vi "ModelCheckNew.vi"(8 "error in (no error)":errorcluster, 9 "ReScanNG":i32, 11 "Data In":T2) -> (0 "error out":errorcluster, 1 "States":T1=enum."Initialize", 2 "ReScanNG":i32, 3 "Data Out":T2)   [LabVIEW 2014]
uses:
  controls/Data1.ctl
  controls/Payjson.ctl
  controls/State.ctl
panel:
  out "Array 2":i32[](array[numeric])
  out "subarray":string[](array[string])
  out "logical AND":bool
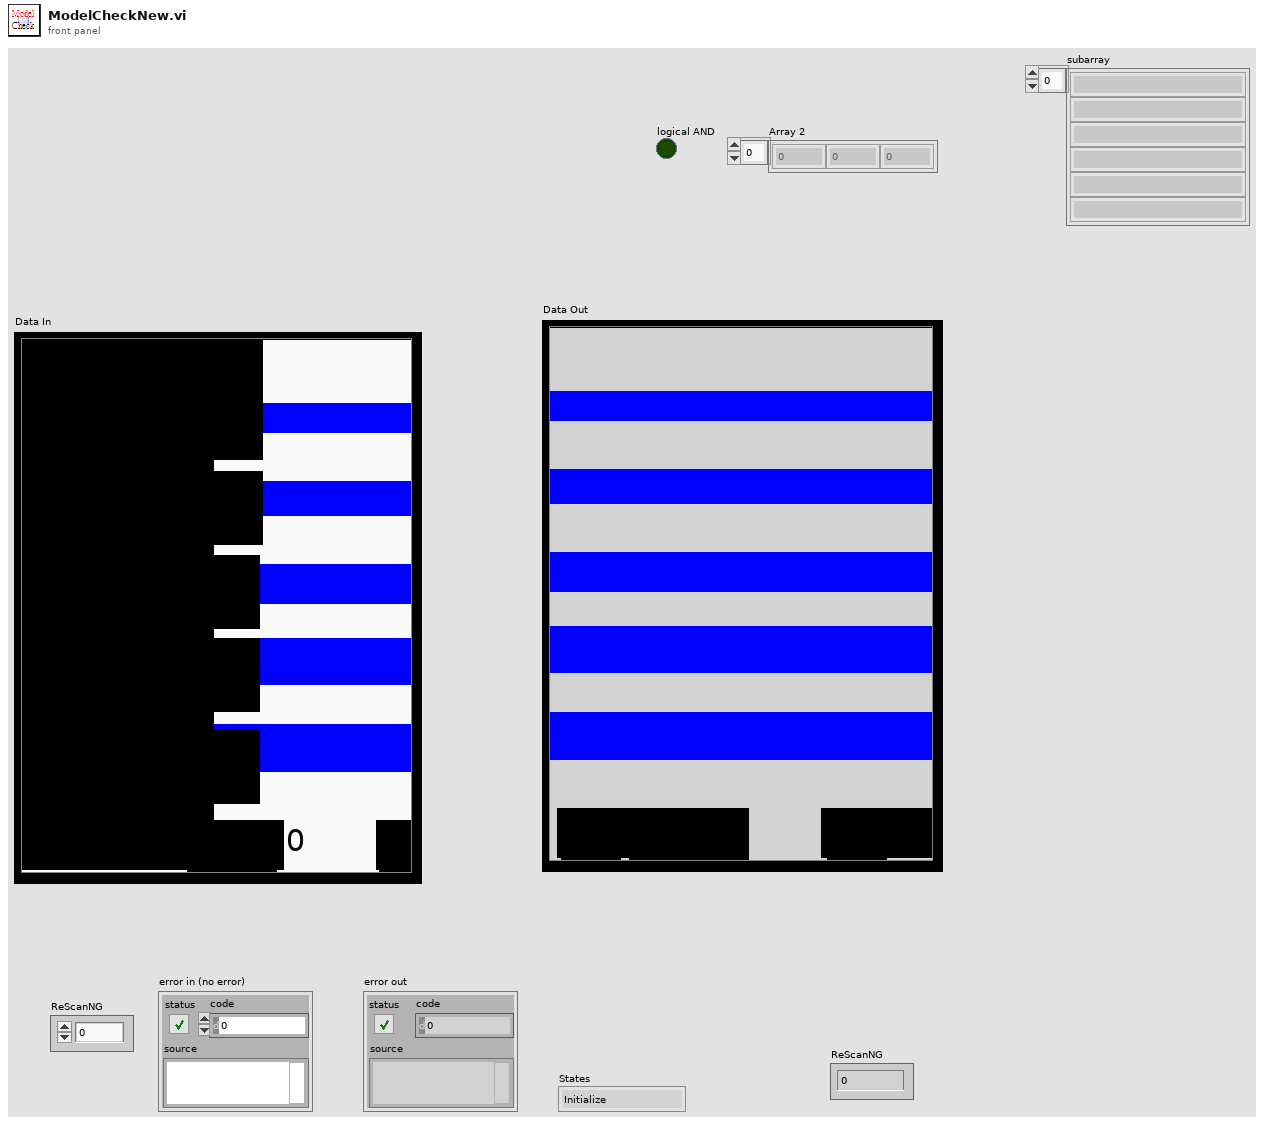
[diagram p1: front panel]
types:
  T1 = typedef "State.ctl" = enum16{"int", "Initalize0", "Initialize", "Wait for Scan", "State 1", "State 2", "NG", "NG1", "OK", "OKNG", "OKNG1", "Exit"}
  T2 = typedef "Data1.ctl" = cluster{"Date":string, "BarCode1":string, "BarCode2":string, "BarCode3":string, "Message":string, "OK Count":u16, "NG Count":u16, "Total Count":u16, "ModelData":string[][], "OK&NG":bool, "COM1":refnum<visa-resource-name>, "COM2":refnum<visa-resource-name>, "IO":i32, "Time":u32, "TCP":refnum<k5>, "TCP 2":refnum<k5>, "COM1 2":refnum<visa-resource-name>, "CheckNum":string, "BarCode1_1":string, "BarCode2_1":string, "BarCode3_1":string, "日期":string, "機種":string, "機號":string, "商品條碼1":string, "OK_1":string, "OK":string, "NG":string, "NG_1":string, "Total":string, "Total_1":string, "ClaerTime":u32, "Pjson":T3, "LotNo":string[], "CheckParsArray":string[], "BarCode4":string, "BarCode4_1":string, "商品條碼2":string, "BarCode5":string, "BarCode5_1":string, "商品條碼3":string, "ReScanNG":i32, "NGTimeCT":u32}
  T3 = typedef "Payjson.ctl" = cluster{"DEPT":string, "LINE":string, "STANO":string, "WORKNO":string, "PRODSN":string, "COMPNTID":string, "COMPNTLOT":string, "COMPNTSN":string, "USEDQTY":i16, "OPDATE":string, "OPUSER":string, "RECVDATE":string, "MMODU":string}[]
  T4 = cluster{"DEPT":string, "LINE":string, "STANO":string, "WORKNO":string, "PRODSN":string, "COMPNTID":string, "COMPNTLOT":string, "COMPNTSN":string, "USEDQTY":i16, "OPDATE":string, "OPUSER":string, "RECVDATE":string, "MMODU":string}
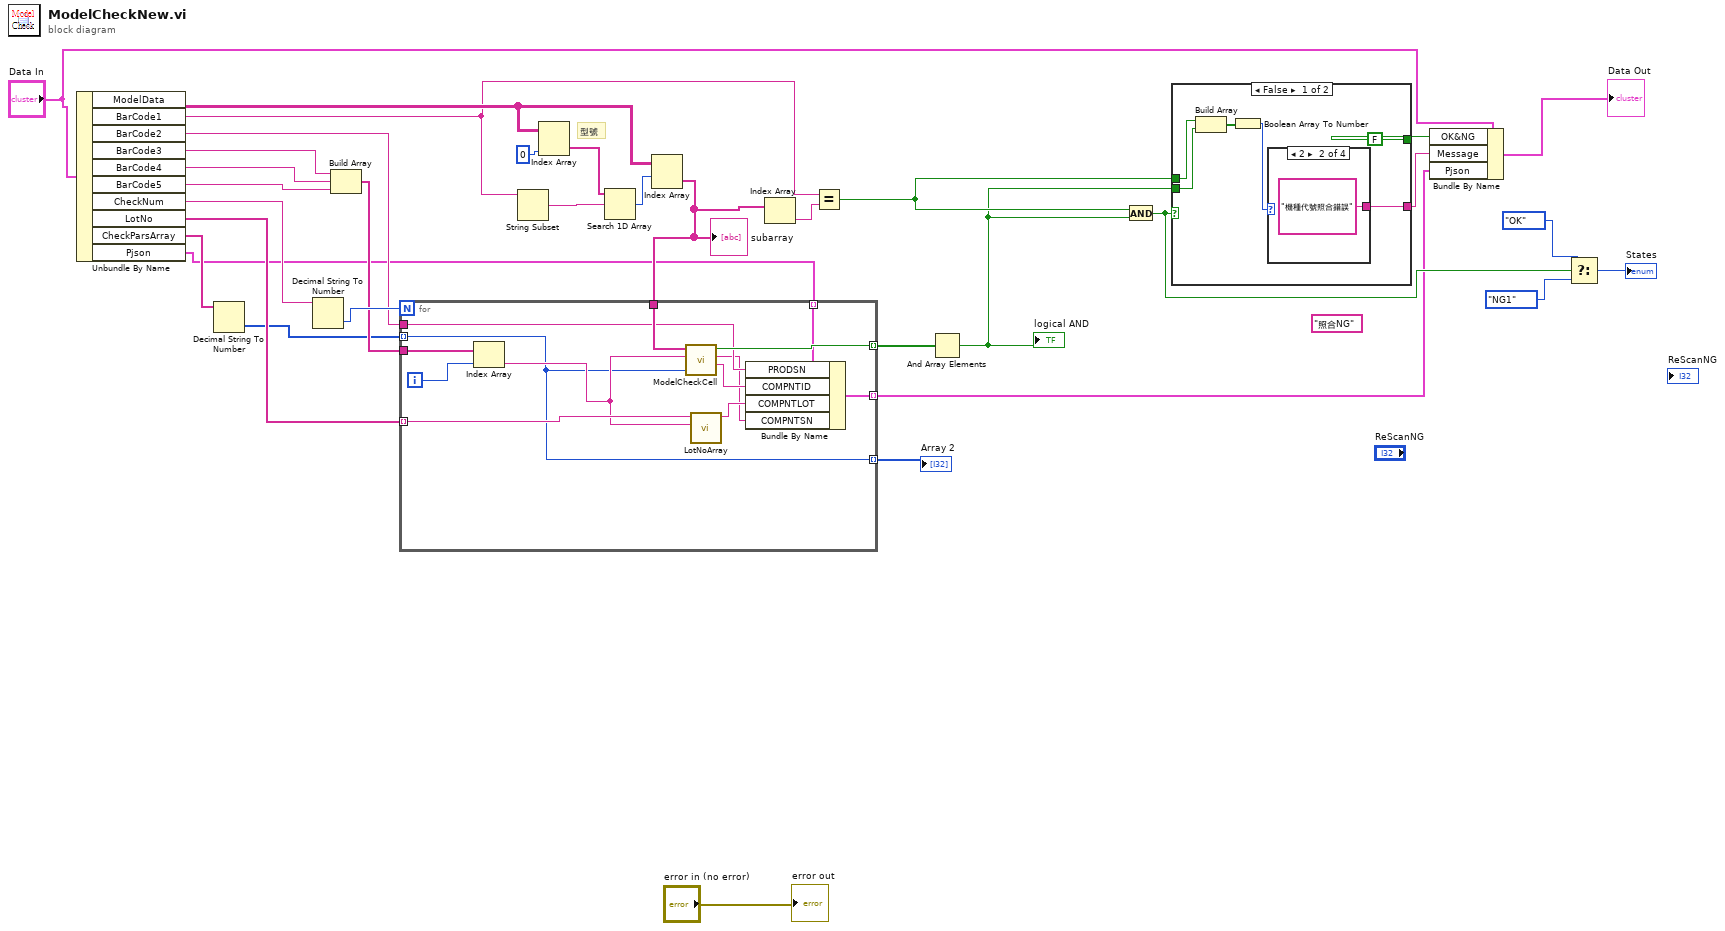
[diagram p0: block diagram]
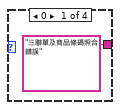
[diagram p2: hidden frame]
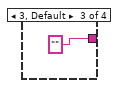
[diagram p3: hidden frame]
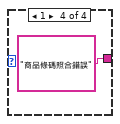
[diagram p4: hidden frame]
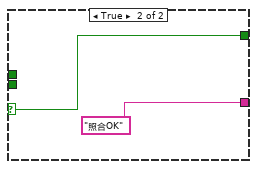
[diagram p5: hidden frame]
diagram:
  (unwired) "照合NG" ("Message")
  # "型號"
  n1 = Unbundle By Name("Data In") -> ("ModelData"=w31:string[][], "BarCode1"=w22:string, "BarCode2"=w3:string, "BarCode3"=w16:string, "BarCode4"=w15:string, "BarCode5"=w14:string, "CheckNum"=w13:string, "LotNo"=w9:string[], "CheckParsArray"=w6:string[], "Pjson"=w2:T3)
  n2 = Decimal String To Number(string=w6) -> (number=w5:i32[])  [unwired: 2 in, 1 out]
  n3 = Decimal String To Number(string=w13) -> (number=w12:i32)  [unwired: 2 in, 1 out]
  n4 = Build Array(w16, w15, w14) -> (w11:string[])
  n5 = String Subset(string=w22) -> (substring=w27:string)  [unwired: 2 in]
  n6 = Index Array(array=w31, index (col)=0 ("disabled index (col)")) -> (element=w32:string[])  [unwired: 1 in]
  n7 = Search 1D Array(1D array=w32, element=w27) -> (index of element=w26:i32)  [unwired: 1 in]
  n8 = Index Array(array=w31, index (row)=w26) -> (element=w10:string[])  [unwired: 1 in]
  "subarray" <- w10
  n9 = for {
    N: w12 -> [_]
    tunnel: w11 -> [w46]
    tunnel: w10 -> [w44]
    tunnel: w9 -> [w43] mode=indexing
    tunnel: [w42] -> w8 mode=indexing
    tunnel: w5 -> [w40] mode=indexing
    tunnel: [w40] -> w4 mode=indexing
    tunnel: w3 -> [w38]
    tunnel: w2 -> [w39] mode=indexing
    tunnel: [w34] -> w1 mode=indexing
    i -> [w45]
    n10 = Index Array(array=w46, index=w45) -> (element=w41:string)
    n11 = call "ModelCheckCell.vi"("checkpars"=w40, "COMPNTSN_in"=w41, "ModelCheckArray"=w44) -> ("COMPNTID"=w37:string, "COMPNTSN"=w35:string, "OK?"=w42:bool)  [unwired: 6 in]
    n12 = call "LotNoArray.vi"("COMPNTSN"=w41, "LotNo"=w43) -> ("COMPNTLOT"=w36:string)  [unwired: 9 in]
    n13 = Bundle By Name(cluster=w39, "PRODSN"=w38, "COMPNTID"=w37, "COMPNTLOT"=w36, "COMPNTSN"=w35) -> (w34:T4)
  }
  "Array 2" <- w4
  n14 = Index Array(array=w10) -> (element=w25:string)  [unwired: 1 in]
  n15 = Equal?(x=w22, y=w25) -> (x = y?=w23:bool)
  n16 = And Array Elements(Boolean array=w8) -> (logical AND=w7:bool)
  "logical AND" <- w7
  n17 = And(x=w23, y=w7) -> (x .and. y?=w19:bool)
  n18 = case shown="False" w19 {
    selector: w19 -> [_ w58]
    tunnel: [FALSE w58] -> w30
    tunnel: [w47 "照合OK" ("Message")] -> w24
    tunnel: w23 -> [w52 _]
    tunnel: w7 -> [w51 _]
    frame False {
      n19 = Build Array(w52, w51) -> (w50:bool[])
      n20 = Boolean Array To Number(Boolean array=w50) -> (number=w48:u32)
      n21 = case shown="2" w48 {
        tunnel: ["三聯單及商品條碼照合錯誤" "機種代號照合錯誤" "" "商品條碼照合錯誤"] -> w47
        frame 0 {
        }
        frame 2 {
        }
        frame 3, Default {
        }
        frame 1 {
        }
      }
    }
    frame True {
    }
  }
  n22 = Bundle By Name(cluster="Data In", "OK&NG"=w30, "Message"=w24, "Pjson"=w1) -> (→"Data Out":T2)
  n23 = Select(t=State."OK" ("States"), s=w19, f=State."NG1" ("States")) -> (s? t:f=→"States":T1)
  "error out" <- "error in (no error)"
